vi "ReentrantVI.vi"() -> (2 "Counter":dbl)   [LabVIEW 2010]
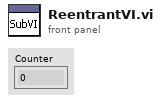
[diagram p1: front panel]
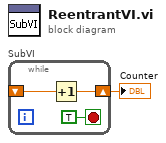
[diagram p0: block diagram]
diagram:
  n1 = while "SubVI" {
    shift-right: [w2] -> w1
    shift-left: _ -> [w3]
    stop <- TRUE stop-if-true
    n2 = Increment(x=w3) -> (x+1=w2:dbl)
  }
  "Counter" <- w1
